vi "Write Frame (Text).vi"(8 "error in (no error)":errorcluster, 9 "timeout (1000 ms)":i32=1000, 10 "Text":string, 11 "Connection.WS":refnum<class "Connection.WS.lvclass">) -> (0 "error out":errorcluster, 3 "Connection.WS":refnum<class "Connection.WS.lvclass">)   [LabVIEW 2013, in "Connection.WS_GOSPL.lvlib" / "Connection.WS.lvclass"]
uses:
  Connection.WS.lvclass
  Websocket Frame Type -- ring.ctl
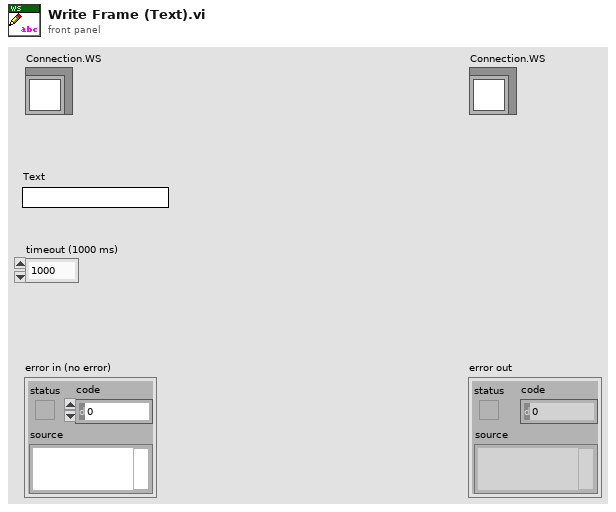
[diagram p1: front panel]
types:
  T1 = typedef "Connection.WS_GOSPL.lvlib/Connection.WS.lvclass/Websocket Frame Type -- ring.ctl" = u8
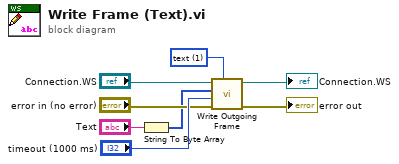
[diagram p0: block diagram]
diagram:
  w8 = T1 1 items=["continuation"=0, "text"=1, "binary"=2, "close"=8, "ping"=9, "pong"=10] ("x")
  n1 = String To Byte Array(string="Text") -> (unsigned byte array=w2:u8[])
  n2 = call "Write Outgoing Frame.vi"("Frame type"=w8, "error in (no error)"="error in (no error)", "timeout ms (2000)"="timeout (1000 ms)", "Bytes"=w2, "Connection.WS"="Connection.WS") -> ("error out"=→"error out":errorcluster, "Connection.WS"=→"Connection.WS":refnum<class "Connection.WS.lvclass">)  [unwired: 5 in]
